vi "JoyStick Global.vi"() -> ()   [LabVIEW 2019]
panel:
  out "Numeric":dbl
  out "Boolean":bool
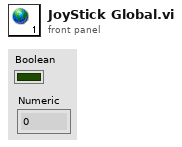
[diagram p1: front panel]
diagram:
